vi "Init Error Task_Manager.vi"(8 "error in (no error)":errorcluster) -> (0 "error out":errorcluster, 3 "Error Task Manager out":refnum<class "Error Task Manager.lvclass">)   [LabVIEW 2013, in "Error Task Manager.lvlib" / "Error Task Manager.lvclass"]
doc: "This Vi Init Task Manager Error"
uses:
  Error Task Manager.lvclass
  Error Task Manager.lvclass/Error Task Manager.ctl
panel:
  in  "Task Manager":errorcluster
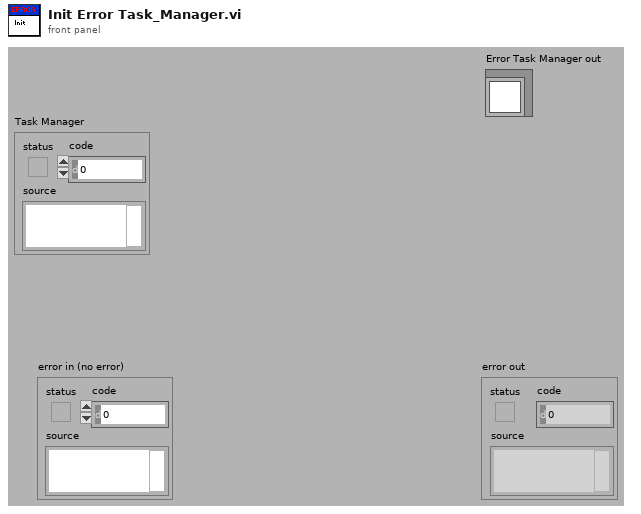
[diagram p1: front panel]
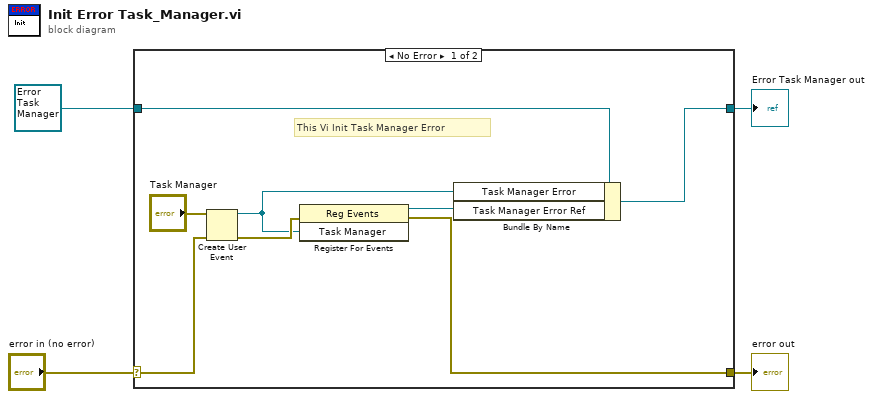
[diagram p0: block diagram]
diagram:
  n1 = case shown="No Error" "error in (no error)" {
    selector: "error in (no error)" -> [w6 w14]
    tunnel: [w5 w14] -> w3
    tunnel: [w7 w13] -> w2
    tunnel: refnum<class "Error Task Manager.lvclass"> refnum ("Error Task Manager.lvlib:Error Task Manager.lvclass") -> [w8 w13]
    frame No Error {
      # "This Vi Init Task Manager Error"
      n2 = Create User Event(user event datatype="Task Manager", error in=w6) -> (user event=w10:refnum<user-event>, error out=w11:errorcluster)
      n3 = register-events(error in=w11, w10) -> (reference out=w9:refnum<event-registration>, error out=w5:errorcluster)  [unwired: 1 in]
      n4 = Bundle By Name(cluster=w8, "Task Manager Error"=w10, "Task Manager Error Ref"=w9) -> (w7:refnum<class "Error Task Manager.lvclass">)
    }
    frame Error {
    }
  }
  "error out" <- w3
  "Error Task Manager out" <- w2
